vi "WriteReadDragPI_YCC.vi"() -> ()   [LabVIEW 2014]
panel:
  in  "Move to Position":bool
  in  "Clear one          all":bool
  in  "Clear Save Position":bool
  in  "Save Position":bool
  in  "Tab Control":enum32{"StandBy", "Drag", "Single WriteRead"}(tab)
  in  "Set ScanRate?":bool
  out "Save Position (um)":dbl[][](array[numeric])
  in  "Clear index (row)":i32
  in  "Move index (row)":i32
  in  "Velocity values":dbl[](array[numeric])=[1000.0, 1000.0, 1000.0] format="%.6f"
  out "XY Position":cluster{"X":dbl, "Y":dbl}[](graph)
  in  "Z  (um)":dbl=50.0 format="%.4f"
  out "Current Z (um)":dbl
  in  "Move Z?":bool
  in  "Adjust to Single Read":bool
  in  "Chang X?":bool
  in  "X Move to (um)":dbl=50.0 format="%_6g"
  in  "Chang Y?":bool
  in  "Y Move to (um)":dbl=50.0 format="%_6g"
  in  "Z Move to (um)":dbl=10.0 format="%_6g"
  in  "Chang Z?":bool
  in  "milliseconds to wait":u32=200
  out "Current Position Z (um)":dbl format="%.4f"
  out "Current Position Y (um)":dbl format="%.4f"
  out "Current Position X (um)":dbl format="%.4f"
  in  "read #":i32=1
  in  "Adjust to cursor":bool=TRUE
  in  "Update ScanRate?":bool
  out "Velocity":dbl[](array[numeric]) format="%.6f"
  in  "Move to (50,50,10) ?":bool
  in  "STOP":bool
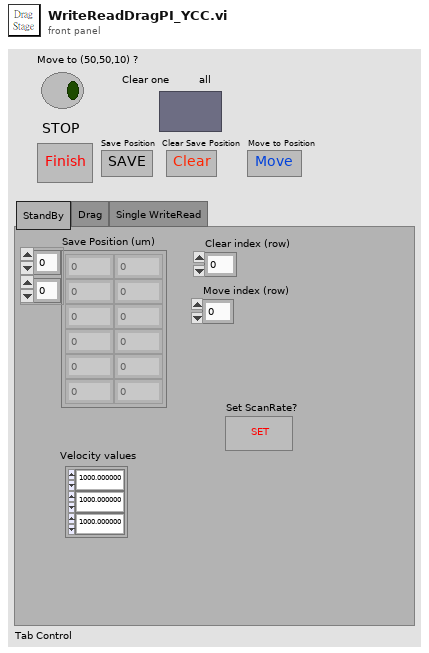
[diagram p1: front panel]
types:
  T1 = enum16{"StandBy", "Drag", "Single WriteRead", "Move to 50,50,50"}
  T2 = typedef "LVPointDoubleTypeDef.ctl" = cluster{"Cursor X":dbl, "Cursor Y":dbl}
  T3 = cluster{"position (um)":dbl, "position (um)":dbl}
  T4 = cluster{"Position wrote to three axis (um)":dbl, "Position wrote to three axis (um)":dbl}
  T5 = cluster{"Real Current Commanded position (um)":dbl, "Real Current Commanded position (um)":dbl}
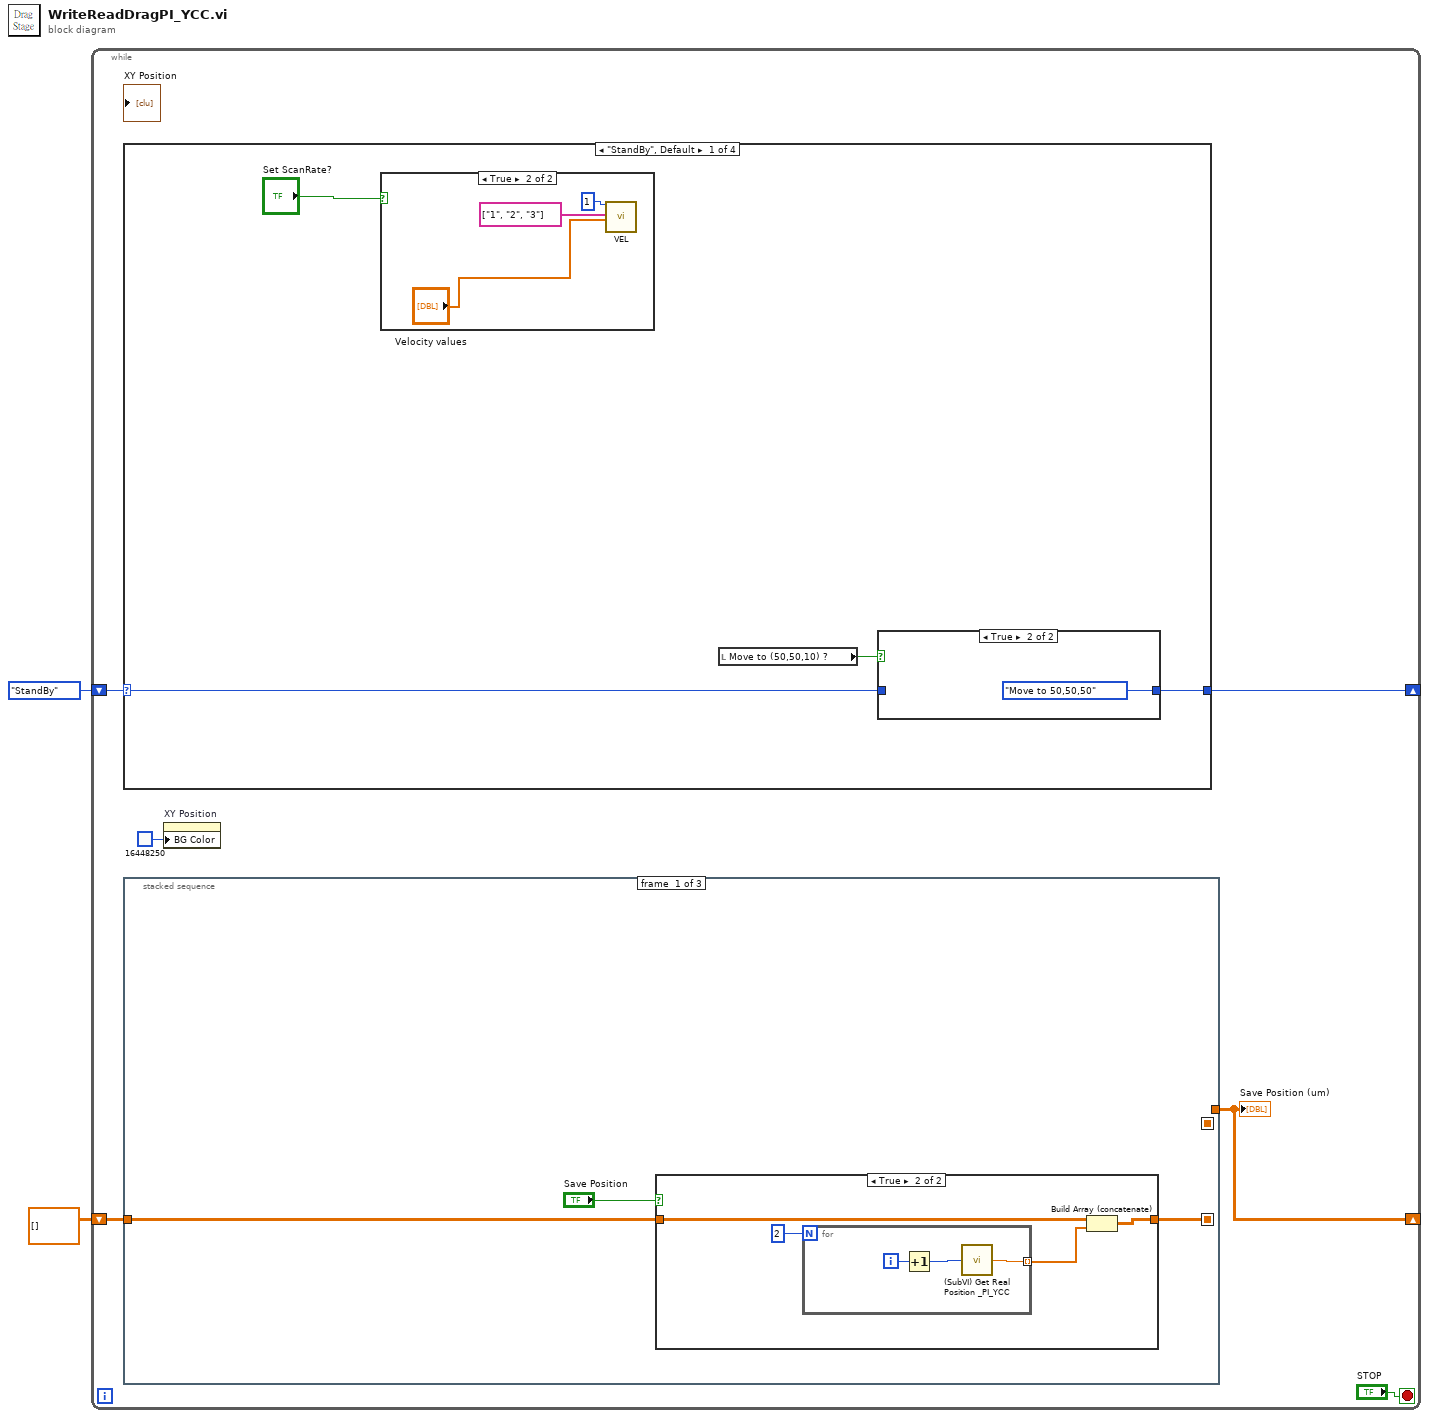
[diagram p0: block diagram]
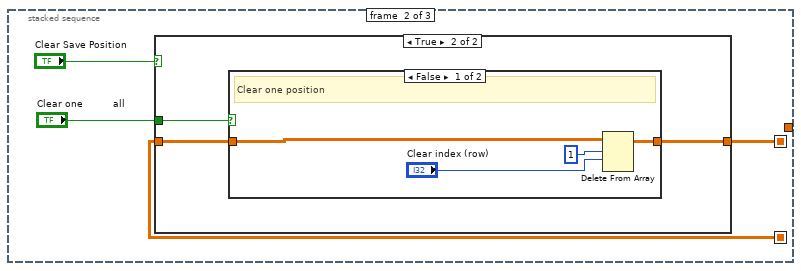
[diagram p3: hidden frame]
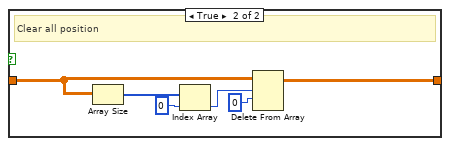
[diagram p5: hidden frame]
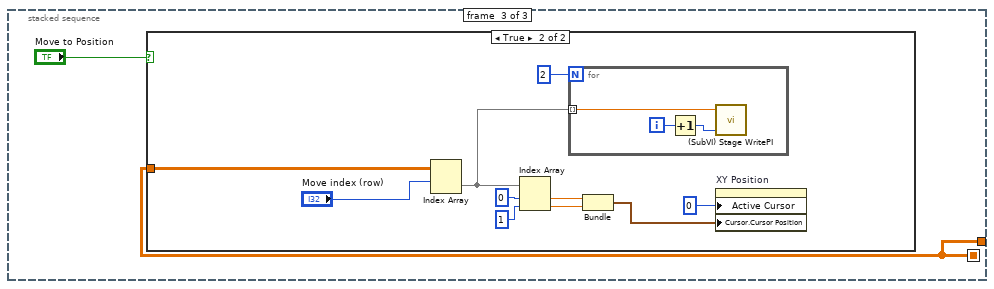
[diagram p6: hidden frame]
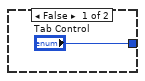
[diagram p9: hidden frame]
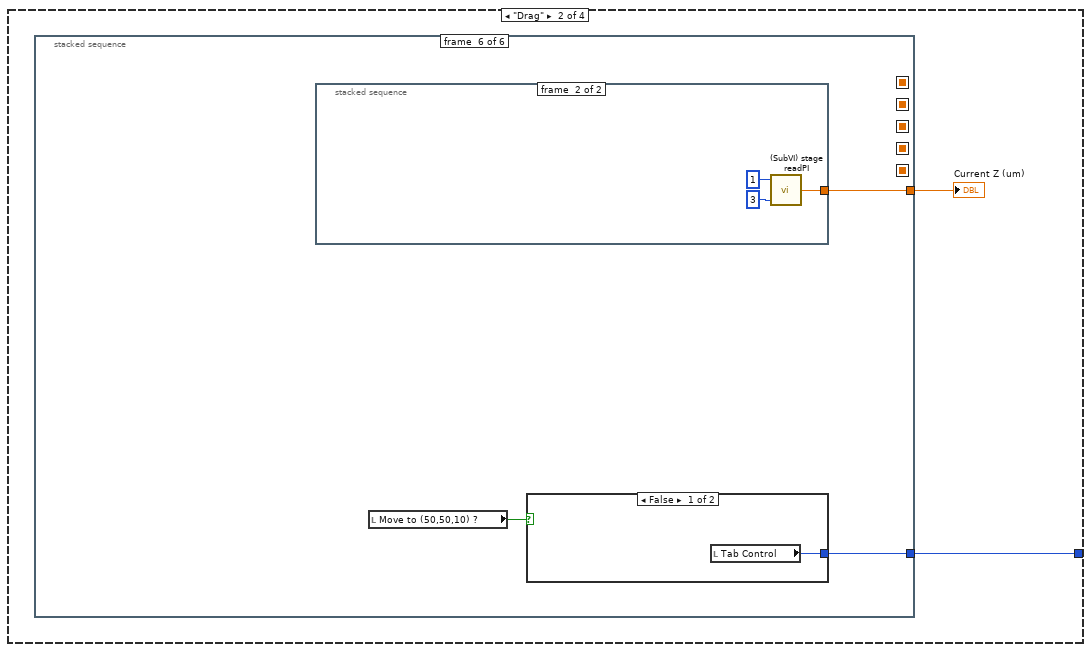
[diagram p10: hidden frame]
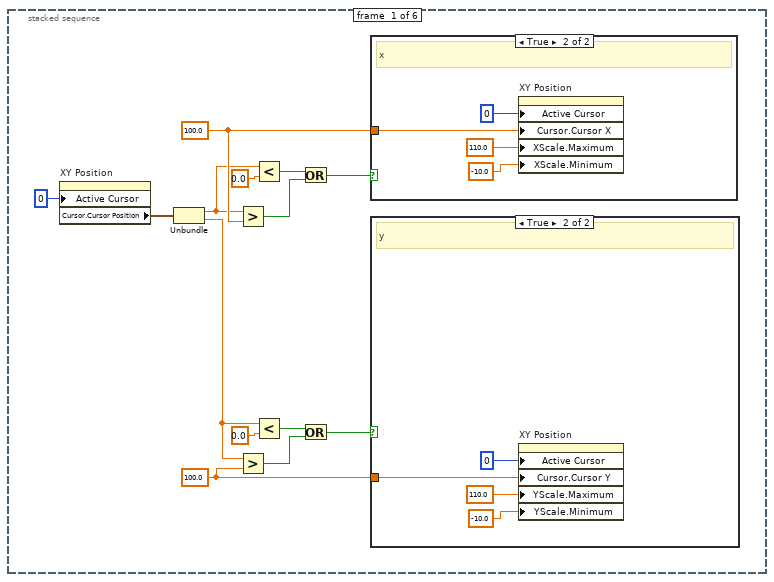
[diagram p11: hidden frame]
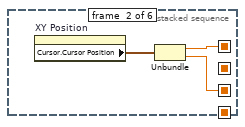
[diagram p14: hidden frame]
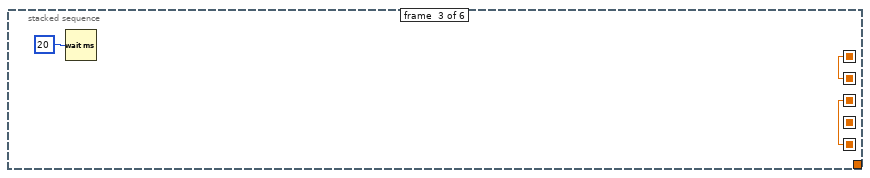
[diagram p15: hidden frame]
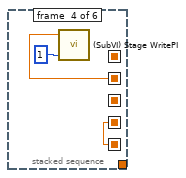
[diagram p16: hidden frame]
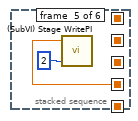
[diagram p17: hidden frame]
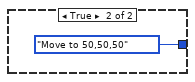
[diagram p18: hidden frame]
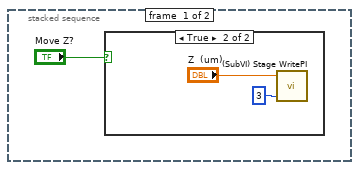
[diagram p19: hidden frame]
diagram:
  n1 = while {
    shift-right: [w8] -> _
    shift-left: T1."StandBy" ("Enum") -> [w6]
    shift-right: [w4] -> _
    shift-left: dbl[][] [] -> [w5]
    stop <- "STOP" stop-if-true
    n2 = case shown="\"StandBy\", Default" w6 {
      selector: w6 -> [w54 _ _ _]
      tunnel: [w55 w62 w108 w160] -> w8
      frame "StandBy", Default {
        n3 = case shown="True" "Set ScanRate?" {
          frame False {
          }
          frame True {
            n4 = call "VEL.vi"("System no."=1, "Axes to set"=string[] ["1", "2", "3"], "Velocity values"="Velocity values") -> ()  [unwired: 15 in, 2 out]
          }
        }
        n5 = local read "Move to (50,50,10) ?"() -> (w56:bool)
        n6 = case shown="True" w56 {
          tunnel: ["Tab Control" T1."Move to 50,50,50" ("Enum")] -> w55
          tunnel: w54 -> [_ _]
          frame False {
          }
          frame True {
          }
        }
      }
      frame "Drag" {
        n7 = stacked-sequence {
          seq-local: [_ w86 _ _ _ _] -> [_ _ w90 _ _ _]
          seq-local: [_ w87 _ _ _ _] -> [_ _ w89 _ _ _]
          seq-local: [_ _ w90 _ _ _] -> [_ _ _ w92 _ _]
          seq-local: [_ _ w89 _ _ _] -> [_ _ _ w93 _ _]
          seq-local: [_ _ _ w92 _ _] -> [_ _ _ _ w95 _]
          tunnel: [_ _ _ _ _ w99] -> w63
          tunnel: [_ _ _ _ _ w97] -> w62
          frame #0 {
            w75 = 100.0 ("y")
            w76 = 100.0 ("y")
            n8 = property on="XY Position" class="XYGraph (strict)"("Active Cursor"=u32 0) -> ("Cursor.Cursor Position"=w77:T2)  [unwired: 2 in, 2 out]
            n9 = Unbundle(w77) -> ("Cursor X"=w73:dbl, "Cursor Y"=w70:dbl)
            n10 = Greater?(x=w73, y=w76) -> (0:w68:bool)
            n11 = Greater?(x=w70, y=w75) -> (0:w65:bool)
            n12 = Less?(x=w73, y=0.0) -> (x < y?=w69:bool)
            n13 = Less?(x=w70, y=0.0) -> (x < y?=w66:bool)
            n14 = Or(x=w69, y=w68) -> (x .or. y?=w67:bool)
            n15 = Or(x=w66, y=w65) -> (x .or. y?=w64:bool)
            n16 = case shown="True" w67 {
              tunnel: w76 -> [_ w85]
              frame False {
              }
              frame True {
                # "x"
                n17 = property on="XY Position" class="XYGraph (strict)"("Active Cursor"=u32 0, "Cursor.Cursor X"=w85, "XScale.Maximum"=110.0 ("X Scale.Range:Maximum"), "XScale.Minimum"=-10.0 ("X Scale.Range:Minimum")) -> ()  [unwired: 2 in, 2 out]
              }
            }
            n18 = case shown="True" w64 {
              tunnel: w75 -> [_ w81]
              frame False {
              }
              frame True {
                # "y"
                n19 = property on="XY Position" class="XYGraph (strict)"("Active Cursor"=u32 0, "Cursor.Cursor Y"=w81, "YScale.Maximum"=110.0 ("X Scale.Range:Maximum"), "YScale.Minimum"=-10.0 ("X Scale.Range:Minimum")) -> ()  [unwired: 2 in, 2 out]
              }
            }
          }
          frame #1 {
            n20 = property on="XY Position" class="XYGraph (strict)"() -> ("Cursor.Cursor Position"=w88:T2)  [unwired: 2 in, 2 out]
            n21 = Unbundle(w88) -> ("Cursor X"=w87:dbl, "Cursor Y"=w86:dbl)
          }
          frame #2 {
            n22 = Wait (ms)(milliseconds to wait=u32 20) -> ()  [unwired: 1 out]
          }
          frame #3 {
            n23 = call "(SubVI) Stage WritePI.vi"("axis"=u32 1, "position"=w93) -> ()  [unwired: 4 in]
          }
          frame #4 {
            n24 = call "(SubVI) Stage WritePI.vi"("axis"=u32 2, "position"=w95) -> ()  [unwired: 4 in]
          }
          frame #5 {
            n25 = stacked-sequence {
              tunnel: [_ w105] -> w99
              frame #0 {
                n26 = case shown="True" "Move Z?" {
                  frame False {
                  }
                  frame True {
                    n27 = call "(SubVI) Stage WritePI.vi"("axis"=u32 3, "position"="Z  (um)") -> ()  [unwired: 4 in]
                  }
                }
              }
              frame #1 {
                n28 = call "(SubVI) stage readPI.vi"("Axis"=u32 3 ("axis"), "read #"=1) -> ("position (um)"=w105:dbl)  [unwired: 3 in]
              }
            }
            n29 = local read "Move to (50,50,10) ?"() -> (w98:bool)
            n30 = case shown="False" w98 {
              tunnel: [w100 T1."Move to 50,50,50" ("Enum")] -> w97
              frame False {
                n31 = local read "Tab Control"() -> (w100:enum32{"StandBy", "Drag", "Single WriteRead"})
              }
              frame True {
              }
            }
          }
        }
        "Current Z (um)" <- w63
      }
      frame "Single WriteRead" {
        n32 = stacked-sequence {
          seq-local: [_ _ _ _ w120 _ _ _ _] -> [_ _ _ _ _ w134 _ _ _]
          seq-local: [_ _ _ _ w119 _ _ _ _] -> [_ _ _ _ _ w133 _ _ _]
          seq-local: [_ _ _ _ _ w134 _ _ _] -> [_ _ _ _ _ _ w138 _ _]
          seq-local: [_ _ _ _ _ w133 _ _ _] -> [_ _ _ _ _ _ w137 _ _]
          tunnel: [_ _ _ _ _ w131 _ _ _] -> w108
          frame #0 {
            # "write x"
            n33 = case shown="True" "Chang X?" {
              frame False {
              }
              frame True {
                n34 = call "(SubVI) Stage WritePI.vi"("axis"=u32 1, "position"="X Move to (um)") -> ()  [unwired: 4 in]
              }
            }
          }
          frame #1 {
            # "write y"
            n35 = case shown="True" "Chang Y?" {
              frame False {
              }
              frame True {
                n36 = call "(SubVI) Stage WritePI.vi"("axis"=u32 2, "position"="Y Move to (um)") -> ()  [unwired: 4 in]
              }
            }
          }
          frame #2 {
            n37 = case shown="True" "Chang Z?" {
              frame False {
              }
              frame True {
                n38 = call "(SubVI) Stage WritePI.vi"("axis"=u32 3, "position"="Z Move to (um)") -> ()  [unwired: 4 in]
              }
            }
          }
          frame #3 {
            n39 = Wait (ms)(milliseconds to wait="milliseconds to wait") -> ()  [unwired: 1 out]
          }
          frame #4 {
            n40 = for {
              N: 3 -> [_]
              tunnel: [w127] -> w125 mode=indexing
              i -> [w130]
              n41 = Increment(x=w130) -> (x+1=w129:i32)
              n42 = call "(SubVI) stage readPI.vi"("Axis"=w129, "read #"="read #") -> ("position (um)"=w127:dbl)  [unwired: 3 in]
            }
            n43 = Index Array(array=w125, index #1=0 ("index"), index #2=1 ("index"), index #3=2 ("index")) -> (element #1=w120:dbl, element #2=w119:dbl, element #3=→"Current Position Z (um)":dbl)
            "Current Position X (um)" <- w120
            "Current Position Y (um)" <- w119
          }
          frame #5 {
            n44 = local read "Move to (50,50,10) ?"() -> (w132:bool)
            n45 = case shown="True" w132 {
              tunnel: [w135 T1."Move to 50,50,50" ("Enum")] -> w131
              frame False {
                n46 = local read "Tab Control"() -> (w135:enum32{"StandBy", "Drag", "Single WriteRead"})
              }
              frame True {
              }
            }
          }
          frame #6 {
            n47 = case shown="True" "Adjust to cursor" {
              tunnel: w138 -> [_ w141]
              tunnel: w137 -> [_ w140]
              frame False {
              }
              frame True {
                n48 = Bundle("position (um)"=w141, "position (um)"=w140) -> (w142:T3)  [unwired: 1 in]
                n49 = property on="XY Position" class="XYGraph (strict)"("Cursor.Cursor Position"=w142) -> ()  [unwired: 2 in, 2 out]
              }
            }
          }
          frame #7 {
            n50 = case shown="True" "Adjust to Single Read" {
              frame False {
              }
              frame True {
                n51 = stacked-sequence {
                  seq-local: [w144 _] -> [_ w155]
                  frame #0 {
                    n52 = for {
                      N: 3 -> [_]
                      tunnel: [w146] -> w144 mode=indexing
                      i -> [w148]
                      n53 = Increment(x=w148) -> (x+1=w147:i32)
                      n54 = call "(SubVI) Get Real Position _PI_YCC.vi"("Axis"=w147) -> ("Real Current Commanded position (um)"=w146:dbl)  [unwired: 4 in]
                    }
                  }
                  frame #1 {
                    n55 = Index Array(array=w155, index #1=0 ("index"), index #2=1 ("index"), index #3=2 ("index")) -> (element #1=w151:dbl, element #2=w150:dbl, element #3=w149:dbl)
                    n56 = local write "X Move to (um)"(w151) -> ()
                    n57 = local write "Y Move to (um)"(w150) -> ()
                    n58 = local write "Z Move to (um)"(w149) -> ()
                  }
                }
              }
            }
          }
          frame #8 {
            n59 = case shown="True" "Update ScanRate?" {
              frame False {
              }
              frame True {
                n60 = call "VEL?.vi"("System no."=1, "All axes?"=TRUE) -> ("Velocity"=→"Velocity":dbl[])  [unwired: 16 in, 1 out]
              }
            }
          }
        }
      }
      frame "Move to 50,50,50" {
        w160 = T1."StandBy" ("Enum")
        n61 = case shown="True" "Move to (50,50,10) ?" {
          frame False {
          }
          frame True {
            n62 = stacked-sequence {
              frame #0 {
                n63 = call "VEL.vi"("System no."=1, "Axes to set"=string[] ["1", "2", "3"], "Velocity values"=dbl[] [1000.0, 1000.0, 1000.0]) -> ()  [unwired: 15 in, 2 out]
              }
              frame #1 {
                n64 = call "(SubVI) Three Axises Move to MiddlePI_YCC.vi"() -> ()  [unwired: 5 in]
              }
              frame #2 {
                w166 = 50.0 ("Position wrote to three axis (um)")
                n65 = Bundle("Position wrote to three axis (um)"=w166, "Position wrote to three axis (um)"=w166) -> (w165:T4)  [unwired: 1 in]
                n66 = property on="XY Position" class="XYGraph (strict)"("Cursor.Cursor Position"=w165) -> ()  [unwired: 2 in, 2 out]
                n67 = Wait (ms)(milliseconds to wait=u32 10) -> ()  [unwired: 1 out]
              }
            }
          }
        }
        n68 = local write "Tab Control"(w160) -> ()
      }
    }
    n69 = stacked-sequence {
      seq-local: [w9 _ _] -> [_ w21 _]
      seq-local: [_ w22 _] -> [_ _ w39]
      tunnel: w5 -> [w10 _ _]
      tunnel: [_ _ w39] -> w4
      frame #0 {
        n70 = case shown="True" "Save Position" {
          tunnel: [w12 w14] -> w9
          tunnel: w10 -> [w12 w13]
          frame False {
          }
          frame True {
            n71 = for {
              N: 2 -> [_]
              tunnel: [w17] -> w15 mode=indexing
              i -> [w19]
              n72 = Increment(x=w19) -> (x+1=w18:i32)
              n73 = call "(SubVI) Get Real Position _PI_YCC.vi"("Axis"=w18) -> ("Real Current Commanded position (um)"=w17:dbl)  [unwired: 4 in]
            }
            n74 = Build Array (concatenate)(w13, w15) -> (w14:dbl[][])
          }
        }
      }
      frame #1 {
        n75 = case shown="True" "Clear Save Position" {
          tunnel: [w24 w25] -> w22
          tunnel: w21 -> [w24 w26]
          tunnel: "Clear one          all" -> [_ w27]
          frame False {
          }
          frame True {
            n76 = case shown="False" w27 {
              tunnel: w26 -> [w31 w37]
              tunnel: [w29 w32] -> w25
              frame False {
                # "Clear one position"
                n77 = Delete From Array(array=w31, length=1, index (row)="Clear index (row)") -> (array with subset deleted=w29:dbl[][])  [unwired: 1 in, 1 out]
              }
              frame True {
                # "Clear all position"
                n78 = Array Size(array=w37) -> (size(s)=w36:i32[])
                n79 = Index Array(array=w36, index=0) -> (element=w34:i32)
                n80 = Delete From Array(array=w37, length=w34, index (row)=0) -> (array with subset deleted=w32:dbl[][])  [unwired: 1 in, 1 out]
              }
            }
          }
        }
      }
      frame #2 {
        n81 = case shown="True" "Move to Position" {
          tunnel: w39 -> [_ w49]
          frame False {
          }
          frame True {
            n82 = Index Array(array=w49, index (row)="Move index (row)") -> (element=w45:dbl[])  [unwired: 1 in]
            n83 = Index Array(array=w45, index #1=0 ("index"), index #2=1 ("index")) -> (element #1=w42:dbl, element #2=w41:dbl)
            n84 = for {
              N: 2 -> [_]
              tunnel: w45 -> [w52] mode=indexing
              i -> [w51]
              n85 = Increment(x=w51) -> (x+1=w50:i32)
              n86 = call "(SubVI) Stage WritePI.vi"("axis"=w50, "position"=w52) -> ()  [unwired: 4 in]
            }
            n87 = Bundle("Real Current Commanded position (um)"=w42, "Real Current Commanded position (um)"=w41) -> (w40:T5)  [unwired: 1 in]
            n88 = property on="XY Position" class="XYGraph (strict)"("Active Cursor"=u32 0, "Cursor.Cursor Position"=w40) -> ()  [unwired: 2 in, 2 out]
          }
        }
      }
    }
    "Save Position (um)" <- w4
    n89 = property on="XY Position" class="XYGraph (strict)"("BG Color"=u32 16448250) -> ()  [unwired: 2 in, 2 out]
  }
